vi "WriteTDMSTest1.vi"() -> ()   [LabVIEW 2016]
panel:
  out "Experiment Description 2":T1={"Sample Description"={"sample name"="SA01234.A", "device"="SA01234.A.20180713", "user"="patrick", "project"="graphene", "description"="sketch SET", "sample GUID"="3EAEE46B-2F5E-4712-8AE3-C241FD138412"}, "Experiment Description"={"folder name"="G:\\data\\graphene\\SA01234.A.20180713", "user description"="sweep Vsg as a function of B", "experiment GUID"="30E3DD13-C39C-4090-BB9A-3764BBD20948", "loop info (?)"=""}, "Krohn-Hite"={"Krohn-Hite Channel Array"=[{"channel"="Channel 1", "input config"="Differential", "gain"=100, "shunt resistor"=50, "input coupling"="", "filter"=""}, {"channel"="Channel 2", "input config"="Differential", "gain"=10, "shunt resistor"=50, "input coupling"="", "filter"=""}, {"channel"="Channel 3", "input config"="SE+ (-gnd)", "gain"=10, "shunt resistor"=0, "input coupling"="", "filter"=""}, {"channel"="Channel 4", "input config"="SE+ (-gnd)", "gain"=10, "shunt resistor"=0, "input coupling"="", "filter"=""}, {"channel"="Channel 5", "input config"="SE+ (-gnd)", "gain"=10, "shunt resistor"=0, "input coupling"="", "filter"=""}]}, "Lockin"={"Lockin AO"={"Lockin AO Channel Array"=[{"name"="0", "amplitude"=0.0, "DC offset"=0.0, "frequency"=13.0, "phase"=0.0, "function"="Sine"}, {"name"="1", "amplitude"=0.0, "DC offset"=0.0, "frequency"=13.0, "phase"=0.0, "function"="Sine"}, {"name"="2", "amplitude"=0.0, "DC offset"=0.0, "frequency"=13.0, "phase"=0.0, "function"="Sine"}, {"name"="3", "amplitude"=0.0, "DC offset"=0.0, "frequency"=13.0, "phase"=0.0, "function"="Sine"}, {"name"="4", "amplitude"=0.0, "DC offset"=0.0, "frequency"=13.0, "phase"=0.0, "function"="Sine"}, {"name"="5", "amplitude"=0.0, "DC offset"=0.0, "frequency"=13.0, "phase"=0.0, "function"="Sine"}, {"name"="6", "amplitude"=0.0, "DC offset"=0.0, "frequency"=13.0, "phase"=0.0, "function"="Sine"}, {"name"="7", "amplitude"=0.0, "DC offset"=0.0, "frequency"=13.0, "phase"=0.0, "function"="Sine"}]}, "Lockin AI"={"Lockin AI Array"=[{"KH Channel"="Channel 1", "AI Channel"="0"}, {"KH Channel"="Channel 2", "AI Channel"="1"}, {"KH Channel"="Channel 3", "AI Channel"="2"}, {"KH Channel"="Channel 4", "AI Channel"="3"}, {"KH Channel"="Channel 5", "AI Channel"="4"}]}, "Lockin REF"={"Lockin REF Array"=[{"frequency"=13.0, "phase"=0.0}]}}}
  out "date/time string":string="2018-10-02--21-17-20"
  out "current time":timestamp=timestamp(3621359841.3756013 s since 1904-01-01)
  in  "file path":path=path "C:/Users/Patrick/Desktop/TEST/TEST.tdms"
  in  "stop":bool
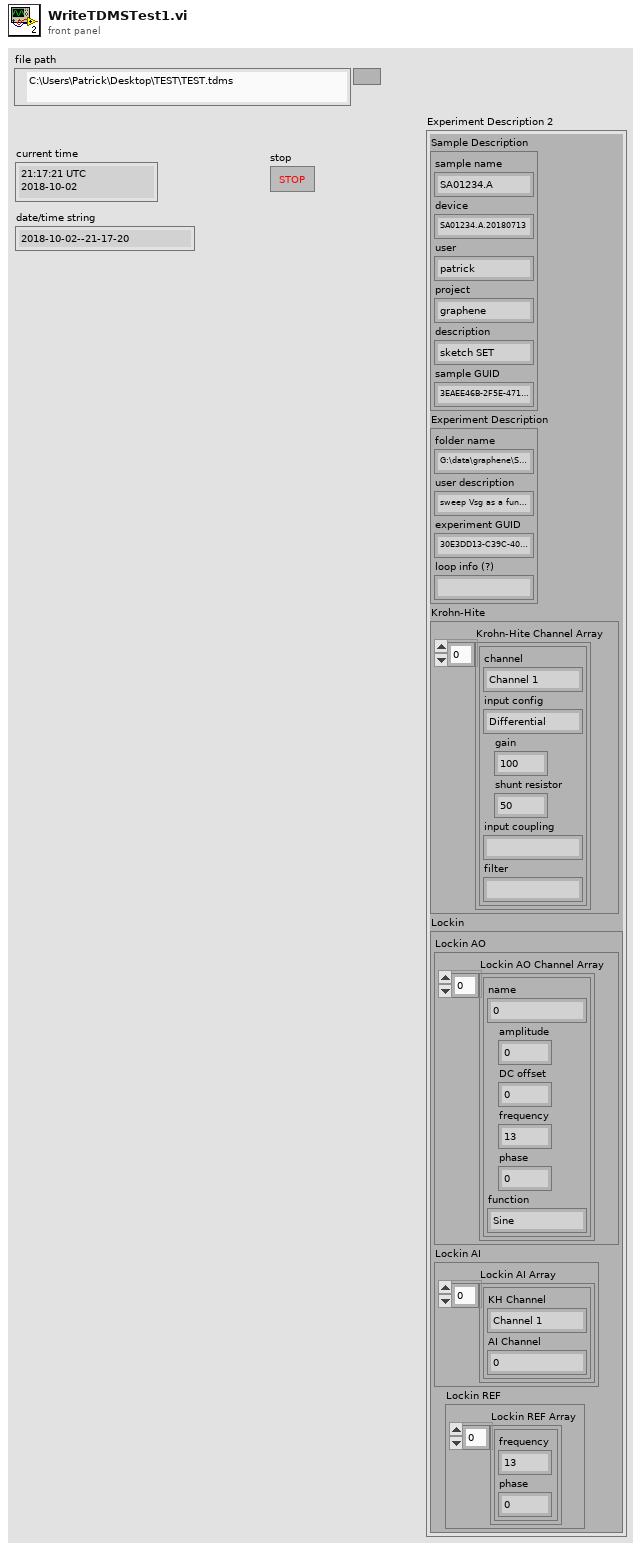
[diagram p1: front panel]
types:
  T1 = cluster{"Sample Description":cluster{"sample name":string, "device":string, "user":string, "project":string, "description":string, "sample GUID":string}, "Experiment Description":cluster{"folder name":string, "user description":string, "experiment GUID":string, "loop info (?)":string}, "Krohn-Hite":cluster{"Krohn-Hite Channel Array":cluster{"channel":string, "input config":string, "gain":i32, "shunt resistor":i32, "input coupling":string, "filter":string}[]}, "Lockin":cluster{"Lockin AO":cluster{"Lockin AO Channel Array":cluster{"name":string, "amplitude":dbl, "DC offset":dbl, "frequency":dbl, "phase":dbl, "function":string}[]}, "Lockin AI":cluster{"Lockin AI Array":cluster{"KH Channel":string, "AI Channel":string}[]}, "Lockin REF":cluster{"Lockin REF Array":cluster{"frequency":dbl, "phase":dbl}[]}}}
  T2 = enum16{"open", "open or create", "create or replace", "create", "open (read-only)"}
  T3 = cluster{"Sample Description":cluster{"name":string, "device":string, "user":string, "project":string, "description":string, "sample GUID":string}, "Experiment Description":cluster{"folder name":string, "user description":string, "experiment GUID":string, "loop info (?)":string}, "Krohn-Hite":cluster{"Krohn-Hite Channel Array":cluster{"channel":string, "input config":string, "gain":i32, "shunt resistor":i32, "input coupling":string, "filter":string}[]}, "Lockin":cluster{"Lockin AO":cluster{"Lockin AO Channel Array":cluster{"name":string, "amplitude":dbl, "DC offset":dbl, "frequency":dbl, "phase":dbl, "function":string}[]}, "Lockin AI":cluster{"Lockin AI Array":cluster{"KH Channel":string, "AI Channel":string}[]}, "Lockin REF":cluster{"Lockin REF Array":cluster{"frequency":dbl, "phase":dbl}[]}}}
  T4 = cluster{"name":string, "device":string, "user":string, "project":string, "description":string, "sample GUID":string}
  T5 = cluster{"folder name":string, "user description":string, "experiment GUID":string, "loop info (?)":string}
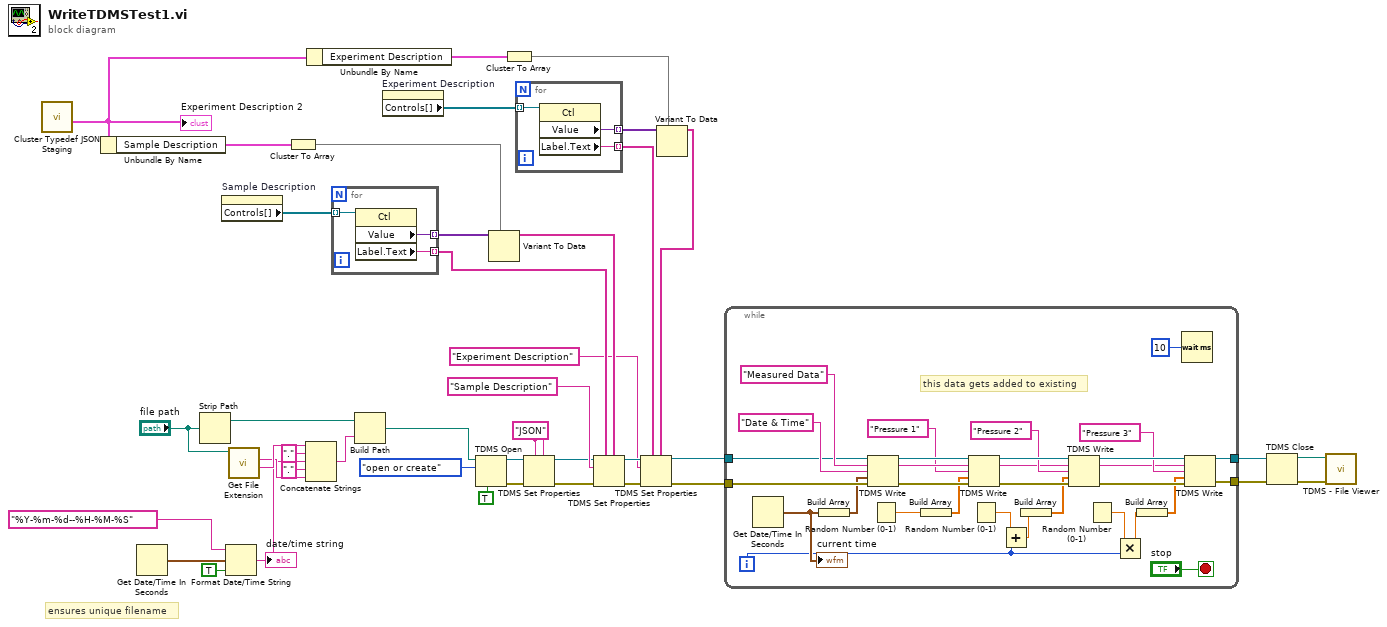
[diagram p0: block diagram]
diagram:
  w1 = "JSON"
  # "ensures unique filename"
  n1 = call "Cluster Typedef JSON Staging.vi"() -> ("Experiment Description 2"=w16:T3)  [unwired: 9 in, 2 out]
  "Experiment Description 2" <- w16
  n2 = Unbundle By Name(w16) -> ("Sample Description"=w21:T4)
  n3 = Get Date/Time In Seconds() -> (seconds since 1Jan1904=w38:timestamp)
  n4 = Strip Path(path="file path") -> (stripped path=w24:path)  [unwired: 1 out]
  n5 = property on="Sample Description" class="Clust (strict)"() -> ("Controls[]"=w42:refnum<vi>[])  [unwired: 2 in, 2 out]
  n6 = Format Date/Time String(time format string (%c)="%Y-%m-%d--%H-%M-%S", seconds (now)=w38, UTC format=TRUE) -> (date/time string=w34:string)
  "date/time string" <- w34
  n7 = call <vilib>:"Get File Extension.vi"("file"="file path") -> ("filename without extension"=w36:string, "lowercase file extension"=w35:string)  [unwired: 6 in, 3 out]
  n8 = Cluster To Array(cluster=w21) -> (array=w40:string[])
  n9 = Concatenate Strings(w36, "." ("string"), w34, "." ("string"), w35) -> (w23:string)
  n10 = Unbundle By Name(w16) -> ("Experiment Description"=w20:T5)
  n11 = for {
    tunnel: w42 -> [w45] mode=indexing
    tunnel: [w44] -> w41 mode=indexing
    tunnel: [w43] -> w13 mode=indexing
    n12 = property class="Ctl"(reference=w45) -> ("Value"=w44:variant, "Label.Text"=w43:string)  [unwired: 1 in, 2 out]
  }
  n13 = Build Path(base path=w24, name or relative path=w23) -> (appended path=w22:path)
  n14 = property on="Experiment Description" class="Clust (strict)"() -> ("Controls[]"=w17:refnum<vi>[])  [unwired: 2 in, 2 out]
  n15 = TDMS Open(6:TRUE ("disable buffering? (T)"), 10:T2."open or create" ("operation (0:open)"), 11:w22) -> (0:w7:errorcluster, 3:w6:refnum<k34>)  [unwired: 4 in]
  n16 = Variant To Data(type=w40, Variant=w41) -> (data=w25:string[])  [unwired: 1 in, 1 out]
  n17 = Cluster To Array(cluster=w20) -> (array=w19:string[])
  n18 = for {
    tunnel: w17 -> [w48] mode=indexing
    tunnel: [w47] -> w18 mode=indexing
    tunnel: [w46] -> w12 mode=indexing
    n19 = property class="Ctl"(reference=w48) -> ("Value"=w47:variant, "Label.Text"=w46:string)  [unwired: 1 in, 2 out]
  }
  n20 = TDMS Set Properties(5:w1, 7:w1, 8:w7, 11:w6) -> (0:w4:errorcluster, 3:w5:refnum<k34>)  [unwired: 2 in, 2 out]
  n21 = TDMS Set Properties(5:w25, 7:w13, 8:w4, 10:"Sample Description" ("group name"), 11:w5) -> (0:w15:errorcluster, 3:w14:refnum<k34>)  [unwired: 1 in, 2 out]
  n22 = Variant To Data(type=w19, Variant=w18) -> (data=w11:string[])  [unwired: 1 in, 1 out]
  n23 = TDMS Set Properties(5:w11, 7:w12, 8:w15, 10:"Experiment Description" ("group name"), 11:w14) -> (0:w3:errorcluster, 3:w2:refnum<k34>)  [unwired: 1 in, 2 out]
  n24 = while {
    tunnel: w3 -> [w76]
    tunnel: [w57] -> w27
    tunnel: [w56] -> w26
    tunnel: w2 -> [w49]
    i -> [w52]
    stop <- "stop" stop-if-true
    # "this data gets added to existing"
    n25 = Get Date/Time In Seconds() -> (seconds since 1Jan1904=w55:timestamp)
    "current time" <- w55
    n26 = Build Array(w55) -> (w74:timestamp[])
    n27 = TDMS Write(0:w49, 5:"Measured Data" ("group name in (Untitled)"), 7:"Date & Time", 9:w74, 11:w76) -> (4:w73:refnum<k34>, 6:w71:string, 15:w72:errorcluster)  [unwired: 1 in, 1 out]
    n28 = Random Number (0-1)() -> (number: 0 to 1=w69:dbl)
    n29 = Build Array(w69) -> (w68:dbl[])
    n30 = TDMS Write(0:w73, 5:w71, 7:"Pressure 1", 9:w68, 11:w72) -> (4:w67:refnum<k34>, 6:w62:string, 15:w66:errorcluster)  [unwired: 1 in, 1 out]
    n31 = Random Number (0-1)() -> (number: 0 to 1=w51:dbl)
    n32 = Add(x=w51, y=w52) -> (x+y=w50:dbl)
    n33 = Build Array(w50) -> (w61:dbl[])
    n34 = TDMS Write(0:w67, 5:w62, 7:"Pressure 2", 9:w61, 11:w66) -> (4:w65:refnum<k34>, 6:w58:string, 15:w64:errorcluster)  [unwired: 1 in, 1 out]
    n35 = Random Number (0-1)() -> (number: 0 to 1=w54:dbl)
    n36 = Multiply(x=w54, y=w52) -> (x*y=w53:dbl)
    n37 = Build Array(w53) -> (w60:dbl[])
    n38 = Wait (ms)(milliseconds to wait=u32 10) -> ()  [unwired: 1 out]
    n39 = TDMS Write(0:w65, 5:w58, 7:"Pressure 3", 9:w60, 11:w64) -> (4:w57:refnum<k34>, 15:w56:errorcluster)  [unwired: 1 in, 2 out]
  }
  n40 = TDMS Close(8:w26, 11:w27) -> (0:w29:errorcluster, 3:w28:path)
  n41 = call <vilib>:"TDMS - File Viewer.vi"("error in (no error)"=w29, "file path"=w28) -> ()  [unwired: 4 in, 2 out]
